vi "CONV 1D Hexidecimal Array to String.vi"(0 "1-D Hexidecimal":u32[](array[numeric]), 1 "Delimiter (,)":string=",") -> (6 "String":string)   [LabVIEW 2012]
doc: "This routine converts a 1-D U32 Hexidecimal Array into a string list. The delimiter may be one or more characters."
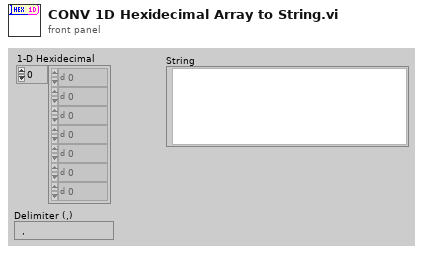
[diagram p1: front panel]
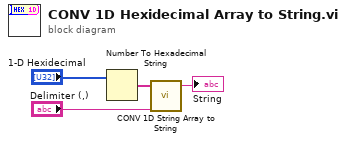
[diagram p0: block diagram]
diagram:
  n1 = Number To Hexadecimal String(2:"1-D Hexidecimal") -> (0:w3:string[])  [unwired: 1 in]
  n2 = call "CONV 1D String Array to String.vi"("1-D String"=w3, "Delimiter (,)"="Delimiter (,)") -> ("String"=→"String":string)  [unwired: 7 in]
